vi "Actor Core.vi"(8 "error in":errorcluster, 11 "Tamagotchi Full Actor in":refnum<class "Tamagotchi Full Actor.lvclass">) -> (0 "error out":errorcluster, 3 "Actor out":refnum<class "Actor.lvclass">)   [LabVIEW 2026, in "Tamagotchi Full Actor.lvclass"]
doc: "<p>(<strong>Filename</strong>: <span class=\"dnl\">Actor Framework.lvlib:Actor.lvclass:Actor Core.vi</span>)</p>\n<p>Receives messages to the actor, reacts to them, and initiates any error handling that may shut the actor down.</p>\n<p>Descendant classes may override this VI to append parallel tasks for the actor to complete while it handles messages. Overrides use the <a href=\"nihelplauncher://docs/csh?context=lvcore_glang_udclass\">Call Parent Class Method</a> node.</p>"
uses:
  Tamagotchi Full Actor.lvclass
  C:/Program Files/National Instruments/LabVIEW 2026/vi.lib/ActorFramework/Actor/Actor.lvclass
  <vilib>/ActorFramework/Actor/Actor.lvclass
  1_QMH/Type Defs/Controls Cluster.ctl
  Tamagotchi Full Actor Messages/Update Cycles Msg/Update Cycles Msg.lvclass
  C:/Program Files/National Instruments/LabVIEW 2026/vi.lib/ActorFramework/Message/Message.lvclass
  Tamagotchi Full Actor Messages/Update UI Msg/Update UI Msg.lvclass
  <vilib>/ActorFramework/Actor/Actor.lvclass/Actor.ctl
  <vilib>/ActorFramework/Message Enqueuer/Message Enqueuer.lvclass/Message Enqueuer.ctl
  <vilib>/ActorFramework/Message Enqueuer/Init from Existing Queue.vi
  <vilib>/ActorFramework/Message Enqueuer/Enqueue.vi
  <vilib>/ActorFramework/Stop Msg/Stop Msg.lvclass
  Tamagotchi Full Actor Messages/Feed Msg/Feed Msg.lvclass
  Tamagotchi Full Actor Messages/Clean Msg/Clean Msg.lvclass
  Tamagotchi Full Actor Messages/Sleep Msg/Sleep Msg.lvclass
  Tamagotchi Full Actor Messages/Spaghetti Msg/Spaghetti Msg.lvclass
  Tamagotchi Full Actor Messages/Broken Arrow Msg/Broken Arrow Msg.lvclass
  Tamagotchi Full Actor Messages/Fixed Bug Msg/Fixed Bug Msg.lvclass
  Tamagotchi Full Actor Messages/Launch Hardware Interface Msg/Launch Hardware Interface Msg.lvclass
  <vilib>/ActorFramework/Message Priority Queue/Priority Enqueue.vi
  <vilib>/ActorFramework/Message Enqueuer/Message Enqueuer.lvclass
  <vilib>/ActorFramework/Actor Framework.lvlib
panel:
  in  "Launch Hardware Interface":bool
  in  "Stop":bool
  out "Age (cycles)":u32
  out "Mood":string
  out "Cleanliness":i16(slide)=100 scale=0.0..100.0
  out "Energy":i16(slide)=100 scale=0.0..100.0
  out "Hunger":i16(slide) scale=0.0..100.0
  in  "Fixed Bug Button":bool
  in  "Broken Arrow Button":bool
  in  "Spagetti Button":bool
  in  "Sleep Button":bool
  in  "Clean Button":bool
  in  "Feed Button":bool
  out "Pict Ring":u16(ring)
  # "Nigel-gotchi (Full Actor)"
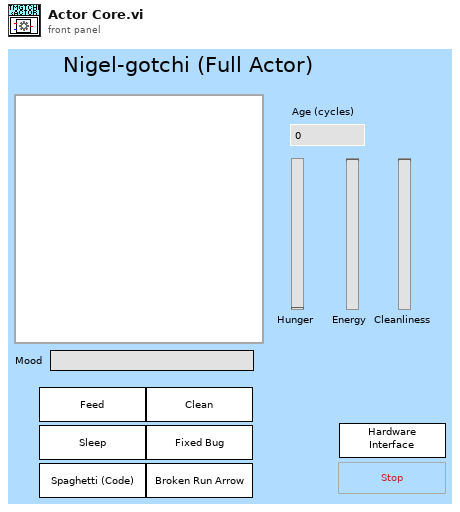
[diagram p1: front panel]
types:
  T1 = typedef "Controls Cluster.ctl" = cluster{"Pict Ring":refnum<vi>, "Mood":refnum<vi>, "Cleanliness":refnum<vi>, "Hunger":refnum<vi>, "Energy":refnum<vi>, "Age (cycles)":refnum<vi>}
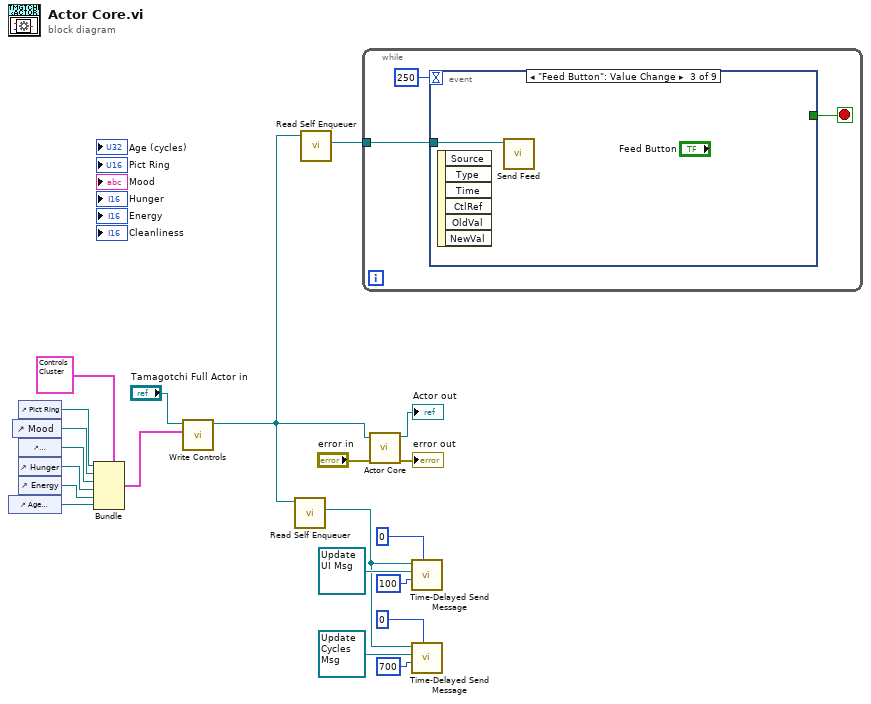
[diagram p0: block diagram]
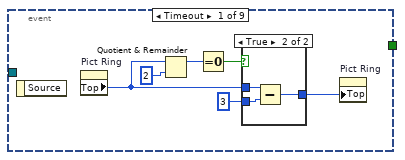
[diagram p2: hidden frame]
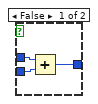
[diagram p3: hidden frame]
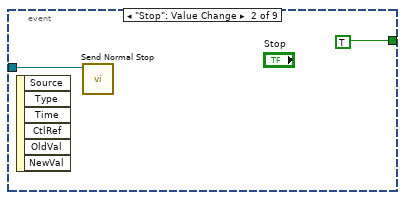
[diagram p4: hidden frame]
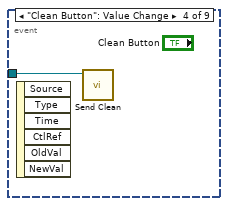
[diagram p5: hidden frame]
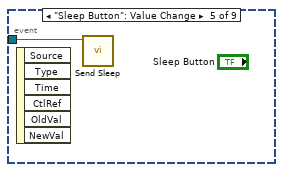
[diagram p6: hidden frame]
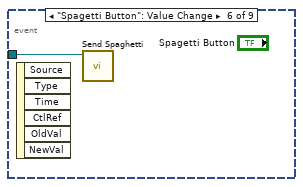
[diagram p7: hidden frame]
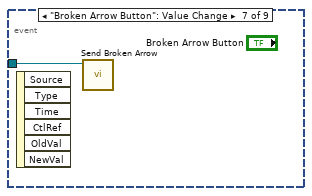
[diagram p8: hidden frame]
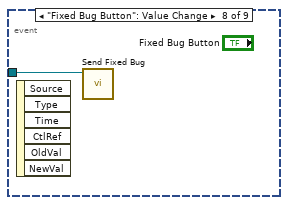
[diagram p9: hidden frame]
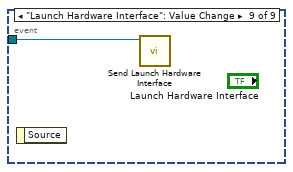
[diagram p10: hidden frame]
diagram:
  n1 = control-ref of="Age (cycles)"() -> (w9:refnum<vi>)
  n2 = control-ref of="Mood"() -> (w13:refnum<vi>)
  n3 = control-ref of="Pict Ring"() -> (w14:refnum<vi>)
  n4 = control-ref of="Cleanliness"() -> (w12:refnum<vi>)
  n5 = control-ref of="Hunger"() -> (w11:refnum<vi>)
  n6 = control-ref of="Energy"() -> (w10:refnum<vi>)
  n7 = Bundle(cluster=T1 {"Pict Ring"=refnum, "Mood"=refnum, "Cleanliness"=refnum, "Hunger"=refnum, "Energy"=refnum, "Age (cycles)"=refnum} ("Controls"), "Pict Ring"=w14, "Mood"=w13, "Cleanliness"=w12, "Hunger"=w11, "Energy"=w10, "Age (cycles)"=w9) -> (w15:T1)
  n8 = call-dynamic "Write Controls.vi"("Controls"=w15, "Nigel Tamagotchi in"="Tamagotchi Full Actor in") -> ("Nigel Tamagotchi out"=w2:refnum<class "Tamagotchi Full Actor.lvclass">)  [unwired: 8 in, 1 out]
  n9 = call <vilib>:"Read Self Enqueuer.vi"("Actor"=w2) -> ("Self Enqueuer"=w1:refnum<class "Message Enqueuer.lvclass">)  [unwired: 10 in]
  n10 = call <vilib>:"Read Self Enqueuer.vi"("Actor"=w2) -> ("Self Enqueuer"=w18:refnum<class "Message Enqueuer.lvclass">)  [unwired: 10 in]
  n11 = while {
    tunnel: w18 -> [w22]
    stop <- w24 stop-if-true
    n12 = event shown="[2] \"Feed Button\": Value Change" {
      selector: _ -> [_ _ _ _ _ _ _ _ _]
      dyn-events: _ -> [_ _ _ _ _ _ _ _ _]
      timeout: 250 -> [_ _ _ _ _ _ _ _ _]
      tunnel: [_ TRUE _ _ _ _ _ _ _] -> w24
      tunnel: w22 -> [_ w38 w39 w40 w41 w42 w43 w44 w45]
      event Timeout {
        n13 = event-data() -> ()  [unwired: 1 in, 1 out]
        n14 = property on="Pict Ring" class="Ring (strict)"() -> ("Top"=w26:i32)  [unwired: 2 in, 2 out]
        n15 = Quotient & Remainder(x=w26, y=2) -> (x-y*floor(x/y)=w29:i32)  [unwired: 1 out]
        n16 = Equal To 0?(x=w29) -> (x = 0?=w30:bool)
        n17 = case shown="True" w30 {
          tunnel: 3 ("y") -> [w33 w36]
          tunnel: [w32 w35] -> w25
          tunnel: w26 -> [w31 w34]
          frame False {
            n18 = Add(x=w31, y=w33) -> (x+y=w32:i32)
          }
          frame True {
            n19 = Subtract(x=w34, y=w36) -> (x-y=w35:i32)
          }
        }
        n20 = property on="Pict Ring" class="Ring (strict)"("Top"=w25) -> ()  [unwired: 2 in, 2 out]
      }
      event "Stop": Value Change {
        n21 = event-data() -> ()  [unwired: 1 in, 6 out]
        n22 = call <vilib>:"Send Normal Stop.vi"("Message Enqueuer"=w38) -> ()  [unwired: 10 in, 1 out]
      }
      event "Feed Button": Value Change {
        n23 = event-data() -> ()  [unwired: 1 in, 6 out]
        n24 = call "Send Feed.vi"("Message Enqueuer"=w39) -> ()  [unwired: 9 in, 2 out]
      }
      event "Clean Button": Value Change {
        n25 = event-data() -> ()  [unwired: 1 in, 6 out]
        n26 = call "Send Clean.vi"("Message Enqueuer"=w40) -> ()  [unwired: 9 in, 2 out]
      }
      event "Sleep Button": Value Change {
        n27 = event-data() -> ()  [unwired: 1 in, 6 out]
        n28 = call "Send Sleep.vi"("Message Enqueuer"=w41) -> ()  [unwired: 9 in, 2 out]
      }
      event "Spagetti Button": Value Change {
        n29 = event-data() -> ()  [unwired: 1 in, 6 out]
        n30 = call "Send Spaghetti.vi"("Message Enqueuer"=w42) -> ()  [unwired: 9 in, 2 out]
      }
      event "Broken Arrow Button": Value Change {
        n31 = event-data() -> ()  [unwired: 1 in, 6 out]
        n32 = call "Send Broken Arrow.vi"("Message Enqueuer"=w43) -> ()  [unwired: 9 in, 2 out]
      }
      event "Fixed Bug Button": Value Change {
        n33 = event-data() -> ()  [unwired: 1 in, 6 out]
        n34 = call "Send Fixed Bug.vi"("Message Enqueuer"=w44) -> ()  [unwired: 9 in, 2 out]
      }
      event "Launch Hardware Interface": Value Change {
        n35 = event-data() -> ()  [unwired: 1 in, 1 out]
        n36 = call "Send Launch Hardware Interface.vi"("Message Enqueuer"=w45) -> ()  [unwired: 9 in, 2 out]
      }
    }
  }
  n37 = call-parent "Actor Core.vi"("error in"="error in", "Actor in"=w2) -> ("error out"=→"error out":errorcluster, "Actor out"=→"Actor out":refnum<class "Actor.lvclass">)  [unwired: 8 in]
  n38 = call <vilib>:"Time-Delayed Send Message.vi"("# Copies (0 = infinite repeat)"=u32 0, "Milliseconds To Wait"=100 ("milliseconds to wait"), "Message"=refnum<class "Update UI Msg.lvclass"> refnum ("Update UI Msg.lvclass"), "Message Enqueuer"=w1) -> ()  [unwired: 6 in, 2 out]
  n39 = call <vilib>:"Time-Delayed Send Message.vi"("# Copies (0 = infinite repeat)"=u32 0, "Milliseconds To Wait"=700 ("milliseconds to wait"), "Message"=refnum<class "Update Cycles Msg.lvclass"> refnum ("Update Cycles Msg.lvclass"), "Message Enqueuer"=w1) -> ()  [unwired: 6 in, 2 out]
